vi "OpenFileSD.vi"(8 "error in (no error)":errorcluster, 10 "File Name":string, 11 "SerialPortRef":T1) -> (0 "error out":errorcluster, 3 "SerialPortRef 2":T1)   [LabVIEW 2016]
uses:
  <vilib>/Rock Robotics/WPI/SerialPort/WPI_SerialPortRef.ctl
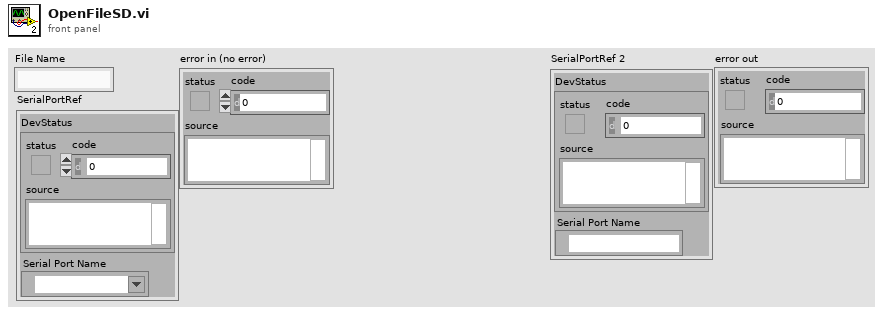
[diagram p1: front panel]
types:
  T1 = typedef "WPI_SerialPortRef.ctl" = cluster{"DevStatus":errorcluster, "Serial Port Name":refnum<visa-resource-name>}
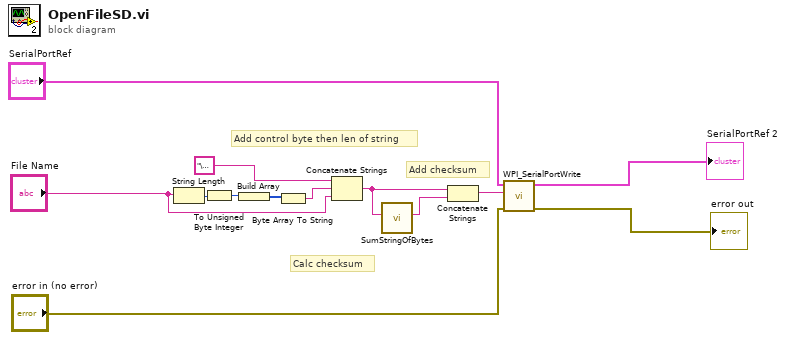
[diagram p0: block diagram]
diagram:
  # "Calc checksum"
  # "Add checksum"
  # "Add control byte then len of string"
  n1 = String Length(string="File Name") -> (length=w7:i32)
  n2 = To Unsigned Byte Integer(number=w7) -> (unsigned 8bit integer=w10:u8)
  n3 = Build Array(w10) -> (w9:u8[])
  n4 = Byte Array To String(unsigned byte array=w9) -> (string=w8:string)
  n5 = Concatenate Strings("\u0003", w8, "File Name") -> (w12:string)
  n6 = call "SumStringOfBytes.vi"("String Of Bytes"=w12) -> ("SumAsString"=w13:string)  [unwired: 10 in]
  n7 = Concatenate Strings(w12, w13) -> (w6:string)
  n8 = call <vilib>:"WPI_SerialPortWrite.vi"("error in (no error)"="error in (no error)", "Buffer"=w6, "SerialPortRef"="SerialPortRef") -> ("error out"=→"error out":errorcluster, "SerialPortRef"=→"SerialPortRef 2":T1)  [unwired: 6 in, 1 out]
